vi "manage breakdown sub.vi"(8 "error in (no error)":errorcluster) -> (0 "error out":errorcluster)   [LabVIEW 2017]
uses:
  <vilib>/addons/database/Connection.llb/DB Tools Open Connec (Path).vi
  <vilib>/addons/database/NI_Database_API.lvlib
panel:
  in  "Action Related To":string(combo)
  in  "Expected Time To Close Action":string
  in  "Submit 2":bool
  in  "Get Reason  2":bool
  in  "CANCEL":bool
  in  "ID":string
  out "Table":string[][][](array[string])
  out "element":string
  out "index of element":i32
  out "data 2":string[][](array[string])
  in  "Select Reason":string(combo)
  in  "Add Action Taken":string
  in  "Shift":string(combo)
  in  "Select Station":string(combo)
  in  "Date":timestamp format="%<%Y-%m-%d>T"
  in  "Select Stakeholder":string(combo)
  # "Manage Breakdown"
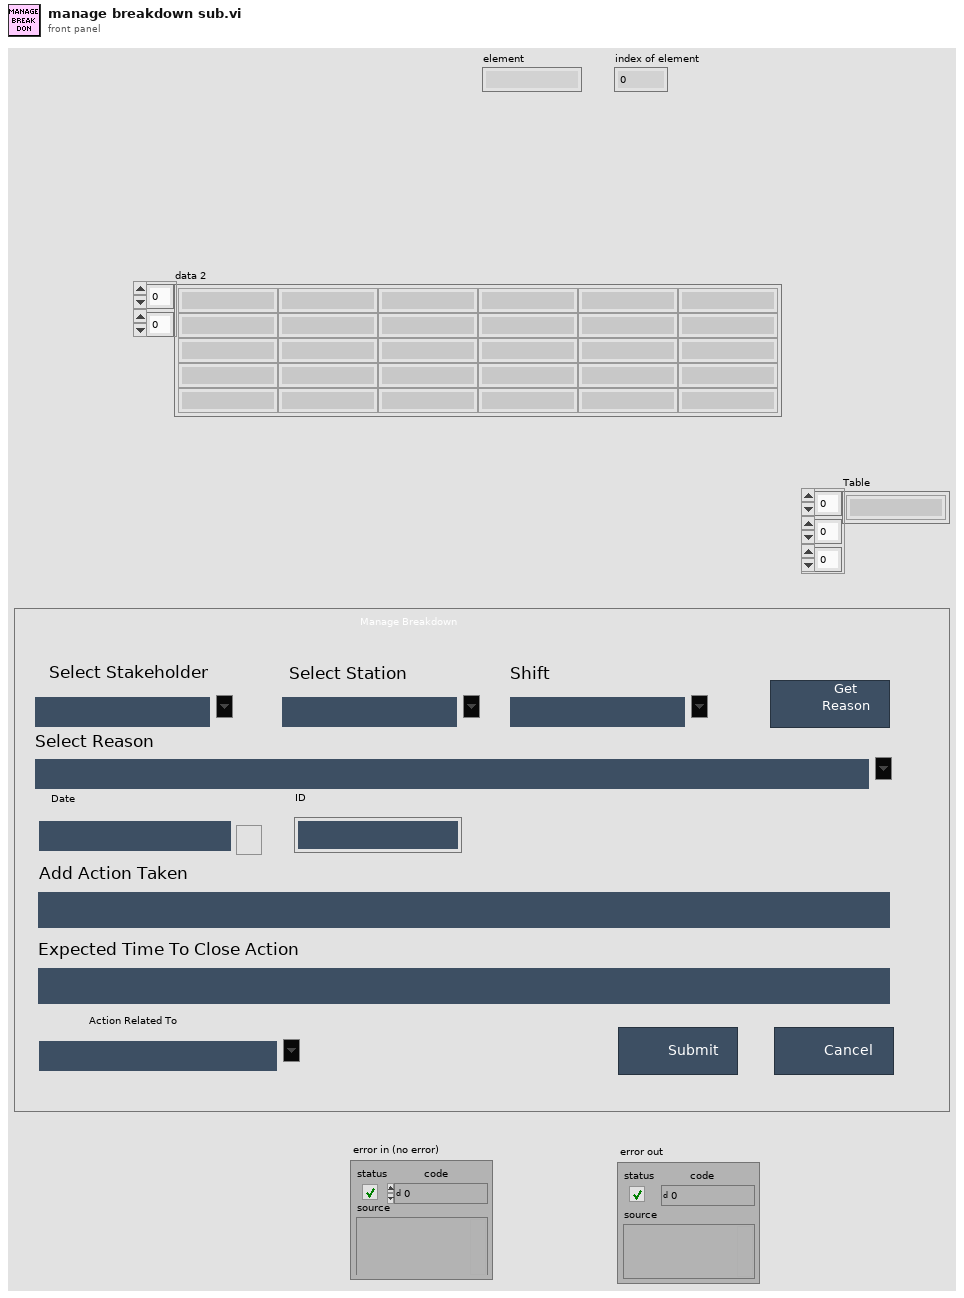
[diagram p1: front panel]
types:
  T1 = typedef "NI_Database_API.lvlib/Conn ObjectReference.ctl" = refnum<k1>
  T2 = enum32{"invalid app kind", "Development System", "Run Time System", "Student Edition", "Embedded LabVIEW", "Evaluation", "Custom"}
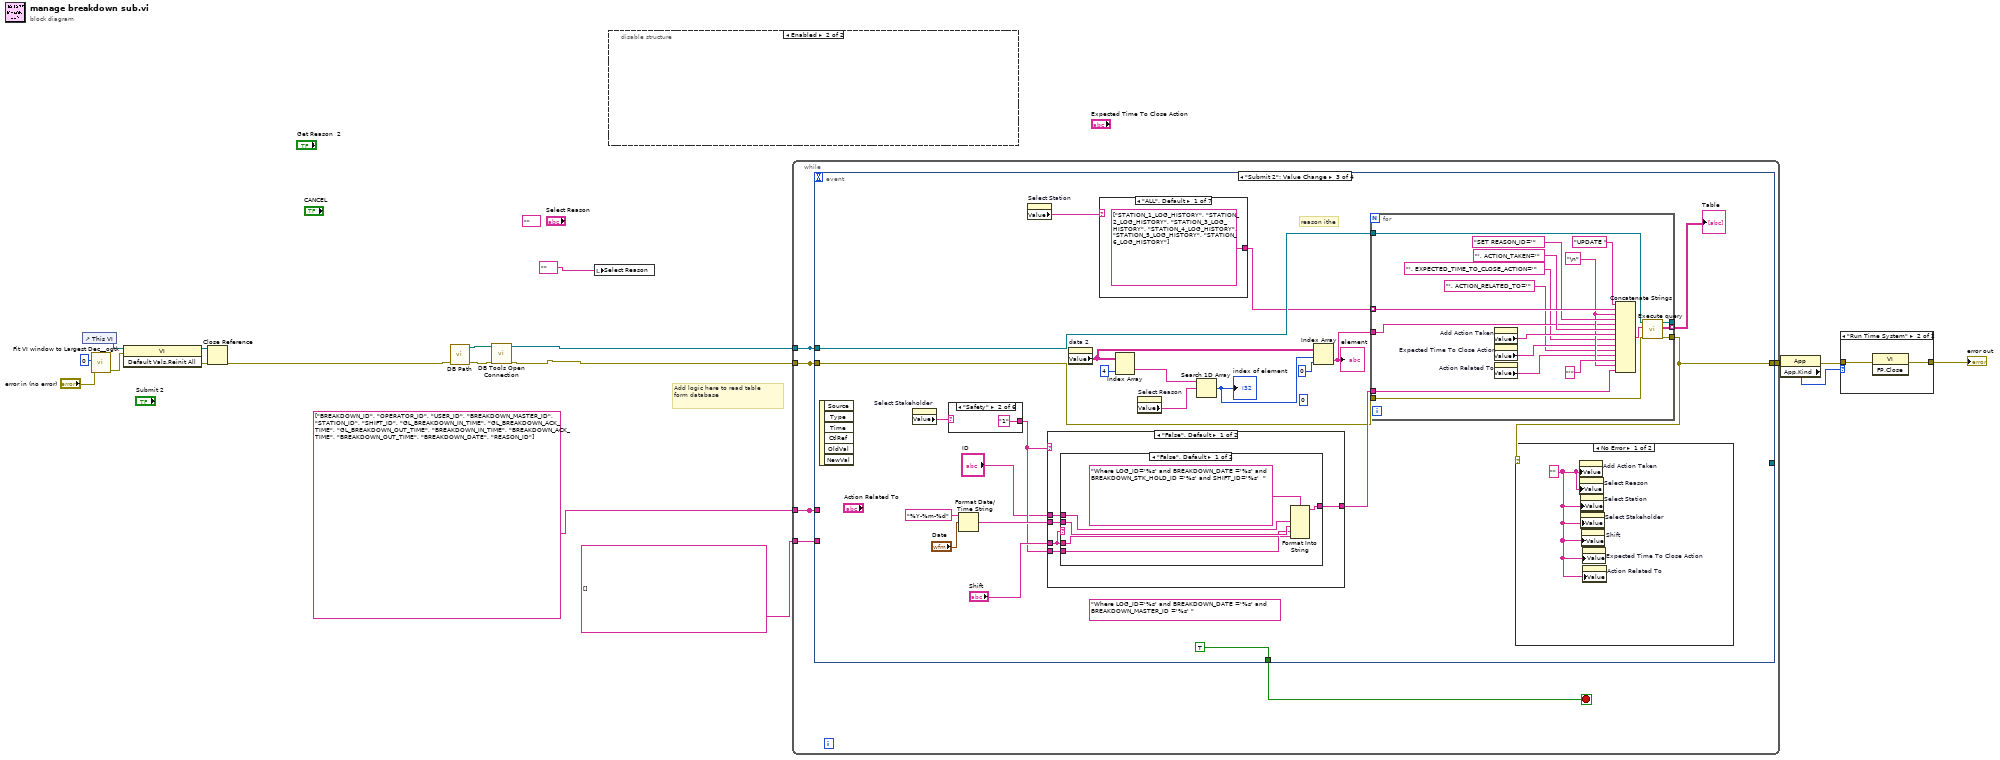
[diagram p0: block diagram]
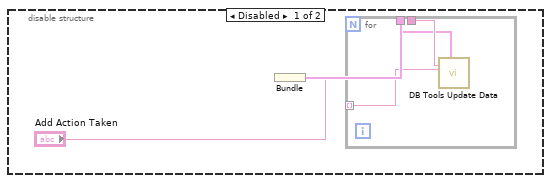
[diagram p2: hidden frame]
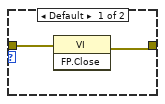
[diagram p3: hidden frame]
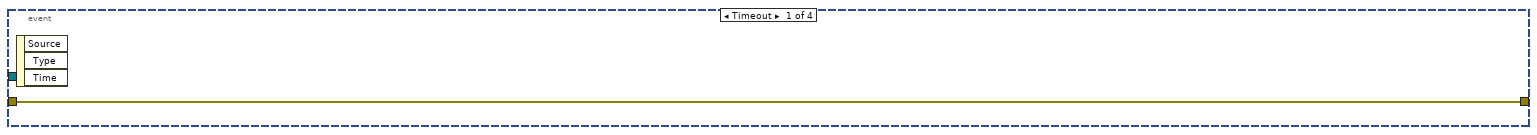
[diagram p4: hidden frame]
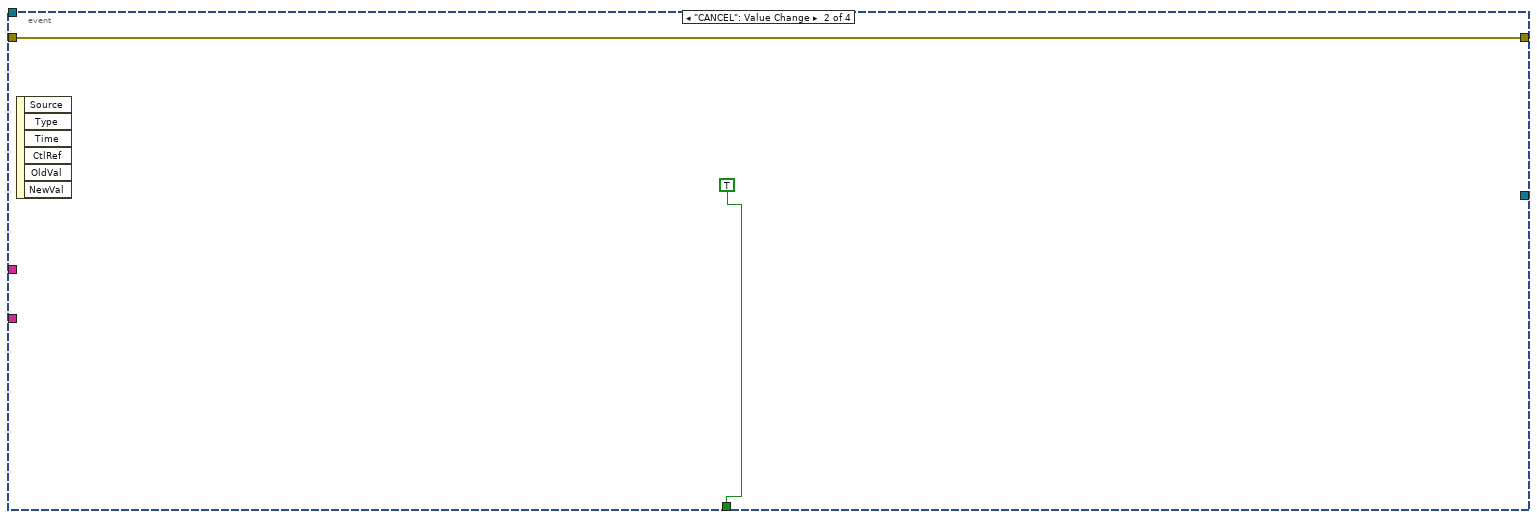
[diagram p5: hidden frame]
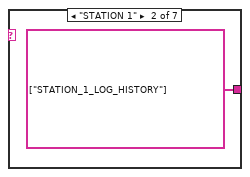
[diagram p6: hidden frame]
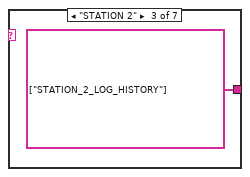
[diagram p7: hidden frame]
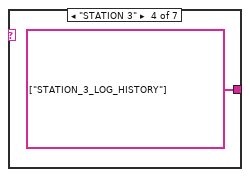
[diagram p8: hidden frame]
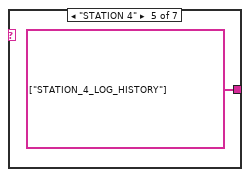
[diagram p9: hidden frame]
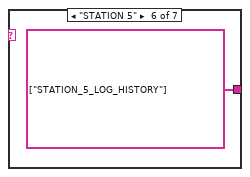
[diagram p10: hidden frame]
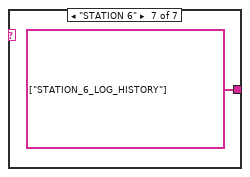
[diagram p11: hidden frame]
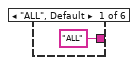
[diagram p13: hidden frame]
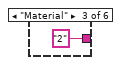
[diagram p14: hidden frame]
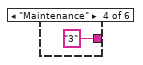
[diagram p15: hidden frame]
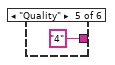
[diagram p16: hidden frame]
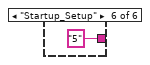
[diagram p17: hidden frame]
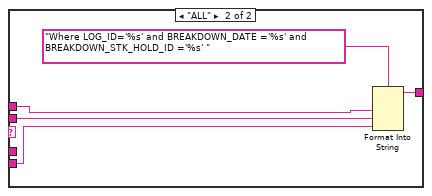
[diagram p18: hidden frame]
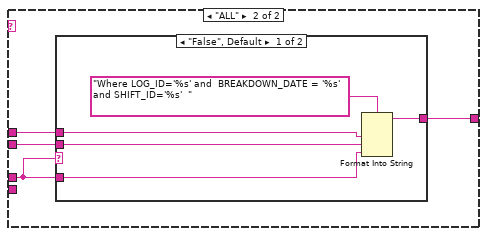
[diagram p19: hidden frame]
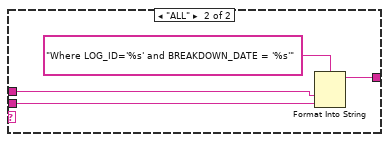
[diagram p20: hidden frame]
diagram:
  (unwired) "" ("Select Reason")
  # "Add logic here to read table\nform database"
  n1 = control-ref of="This VI"() -> (w18:refnum<vi>)
  n2 = call <userlib>:"Fit VI window to Largest Dec__ogtk.vi"("error in (no error)"="error in (no error)", "border spacing (2 px)"=0) -> ("error out"=w10:errorcluster)  [unwired: 4 in, 1 out]
  n3 = invoke class="VI" method="Default Vals.Reinit All"(reference=w18, error in=w10) -> (reference out=w16:refnum<vi>, error out=w17:errorcluster)  [unwired: 1 in, 1 out]
  n4 = Close Reference(reference=w16, error in (no error)=w17) -> (error out=w8:errorcluster)
  n5 = call "DB Path.vi"("error in"=w8) -> ("error out"=w6:errorcluster, "DB Path"=w7:path)  [unwired: 9 in]
  n6 = call-poly <vilib>:"DB Tools Open Connection.vi"("error in (no error)"=w6, "connection information"=w7) -> ("error out"=w5:errorcluster, "connection reference"=w4:T1)  [unwired: 6 in]
  n7 = local write "Select Reason"("" ("Combo Box")) -> ()
  n8 = disable-structure shown="Enabled" {
    frame Disabled {
      n9 = Bundle("Add Action Taken"="Add Action Taken") -> (w20:cluster{"Add Action Taken":string})  [unwired: 1 in]
      n10 = for {
        tunnel: _ -> [w23]
        tunnel: _ -> [w22] mode=indexing
        tunnel: w20 -> [w21]
        n11 = call <vilib>:"DB Tools Update Data.vi"("condition"=w23, "data"=w21, "table"=w22) -> ()  [unwired: 7 in, 2 out]
      }
    }
    frame Enabled {
    }
  }
  n12 = while {
    tunnel: w5 -> [w26]
    tunnel: [w24] -> w12
    tunnel: w4 -> [w27]
    tunnel: string[] ["BREAKDOWN_ID", "OPERATOR_ID", "USER_ID", "BREAKDOWN_MASTER_ID", "STATION_ID", "SHIFT_ID", "GL_BREAKDOWN_IN_TIME", "GL_BREAKDOWN_ACK_TIME", "GL_BREAKDOWN_OUT_TIME", "BREAKDOWN_IN_TIME", "BREAKDOWN_ACK_TIME", "BREAKDOWN_OUT_TIME", "BREAKDOWN_DATE", "REASON_ID"] ("columns") -> [w28]
    tunnel: [w28] -> _
    tunnel: [w26] -> _
    tunnel: [w27] -> _
    tunnel: string[] [] -> [w25]
    stop <- w29 stop-if-true
    n13 = event shown="[2] \"Submit 2\": Value Change" {
      selector: _ -> [_ _ _ _]
      dyn-events: _ -> [_ _ _ _]
      timeout: _ -> [_ _ _ _]
      tunnel: [_ TRUE TRUE _] -> w29
      tunnel: w27 -> [_ _ w40 w131]
      tunnel: w28 -> [_ _ _ _]
      tunnel: w26 -> [w30 w32 w41 w130]
      tunnel: [_ _ _ w129] -> _
      tunnel: w25 -> [_ _ _ _]
      tunnel: [w30 w32 w36 w122] -> w24
      event Timeout {
        n14 = event-data() -> ()  [unwired: 1 in, 3 out]
      }
      event "CANCEL": Value Change {
        n15 = event-data() -> ()  [unwired: 1 in, 6 out]
      }
      event "Submit 2": Value Change {
        (unwired) "Where LOG_ID='%s' and BREAKDOWN_DATE ='%s' and BREAKDOWN_MASTER_ID ='%s' " ("condition")
        (unwired) 0 ("disabled index (col)")
        # "reason ithe"
        n16 = event-data() -> ()  [unwired: 1 in, 6 out]
        n17 = property on="Select Stakeholder" class="CmbBox"() -> ("Value"=w39:string)  [unwired: 2 in, 2 out]
        n18 = case shown="\"Safety\"" w39 {
          tunnel: ["ALL" "1" "2" "3" "4" "5"] -> w38
          frame "ALL", Default {
          }
          frame "Safety" {
          }
          frame "Material" {
          }
          frame "Maintenance" {
          }
          frame "Quality" {
          }
          frame "Startup_Setup" {
          }
        }
        n19 = Format Date/Time String(time format string (%c)="%Y-%m-%d", seconds (now)="Date") -> (date/time string=w47:string)  [unwired: 1 in]
        n20 = property on="Select Station" class="CmbBox"() -> ("Value"=w34:string)  [unwired: 2 in, 2 out]
        n21 = case shown="\"False\", Default" w38 {
          tunnel: [w92 w107] -> w48
          tunnel: w47 -> [w91 w106]
          tunnel: w38 -> [w90 _]
          tunnel: "Shift" -> [w89 w105]
          tunnel: "ID" -> [w88 w104]
          frame "False", Default {
            n22 = case shown="\"False\", Default" w89 {
              tunnel: [w97 w102] -> w92
              tunnel: w91 -> [w96 w101]
              tunnel: w90 -> [w95 w100]
              tunnel: w89 -> [w94 _]
              tunnel: w88 -> [w93 w99]
              frame "False", Default {
                n23 = Format Into String(format string="Where LOG_ID='%s' and BREAKDOWN_DATE ='%s' and BREAKDOWN_STK_HOLD_ID ='%s' and SHIFT_ID='%s'  " ("condition"), w93, w96, w95, w94) -> (resulting string=w97:string)  [unwired: 2 in, 1 out]
              }
              frame "ALL" {
                n24 = Format Into String(format string="Where LOG_ID='%s' and BREAKDOWN_DATE ='%s' and BREAKDOWN_STK_HOLD_ID ='%s' " ("condition"), w99, w101, w100) -> (resulting string=w102:string)  [unwired: 2 in, 1 out]
              }
            }
          }
          frame "ALL" {
            n25 = case shown="\"False\", Default" w105 {
              tunnel: [w111 w115] -> w107
              tunnel: w106 -> [w110 w114]
              tunnel: w105 -> [w109 _]
              tunnel: w104 -> [w108 w113]
              frame "False", Default {
                n26 = Format Into String(format string="Where LOG_ID='%s' and  BREAKDOWN_DATE = '%s' and SHIFT_ID='%s'  " ("condition"), w108, w110, w109) -> (resulting string=w111:string)  [unwired: 2 in, 1 out]
              }
              frame "ALL" {
                n27 = Format Into String(format string="Where LOG_ID='%s' and BREAKDOWN_DATE = '%s'" ("condition"), w113, w114) -> (resulting string=w115:string)  [unwired: 2 in, 1 out]
              }
            }
          }
        }
        n28 = property on="data 2" class="Arr (strict)"() -> ("Value"=w51:string[][])  [unwired: 2 in, 2 out]
        n29 = case shown="\"ALL\", Default" w34 {
          tunnel: [string[] ["STATION_1_LOG_HISTORY", "STATION_2_LOG_HISTORY", "STATION_3_LOG_HISTORY", "STATION_4_LOG_HISTORY", "STATION_5_LOG_HISTORY", "STATION_6_LOG_HISTORY"] string[] ["STATION_1_LOG_HISTORY"] string[] ["STATION_2_LOG_HISTORY"] string[] ["STATION_3_LOG_HISTORY"] string[] ["STATION_4_LOG_HISTORY"] string[] ["STATION_5_LOG_HISTORY"] string[] ["STATION_6_LOG_HISTORY"]] -> w33
          frame "ALL", Default {
          }
          frame "STATION 1" {
          }
          frame "STATION 2" {
          }
          frame "STATION 3" {
          }
          frame "STATION 4" {
          }
          frame "STATION 5" {
          }
          frame "STATION 6" {
          }
        }
        n30 = Index Array(array=w51, index (col)=4 ("disabled index (col)")) -> (element=w49:string[])  [unwired: 1 in]
        n31 = property on="Select Reason" class="CmbBox"() -> ("Value"=w52:string)  [unwired: 2 in, 2 out]
        n32 = Search 1D Array(1D array=w49, element=w52) -> (index of element=w50:i32)  [unwired: 1 in]
        "index of element" <- w50
        n33 = Index Array(array=w51, index (row)=w50, index (col)=0 ("disabled index (col)")) -> (element=w53:string)
        "element" <- w53
        n34 = for {
          tunnel: w33 -> [w85] mode=indexing
          tunnel: w48 -> [w79]
          tunnel: w53 -> [w78]
          tunnel: [w77] -> _
          tunnel: w40 -> [w76]
          tunnel: [w75] -> w36
          tunnel: w41 -> [w74]
          tunnel: [w73] -> w37 mode=indexing
          w80 = "\n" ("string")
          n35 = property on="Add Action Taken" class="Str"() -> ("Value"=w82:string)  [unwired: 2 in, 2 out]
          n36 = property on="Expected Time To Close Action" class="Str"() -> ("Value"=w71:string)  [unwired: 2 in, 2 out]
          n37 = property on="Action Related To" class="CmbBox"() -> ("Value"=w69:string)  [unwired: 2 in, 2 out]
          n38 = Concatenate Strings("UPDATE " ("String"), w85, w80, "SET REASON_ID='" ("string"), w78, "', ACTION_TAKEN='" ("string"), w82, "', EXPECTED_TIME_TO_CLOSE_ACTION='" ("string"), w71, "', ACTION_RELATED_TO='" ("string"), w69, "'" ("string"), w80, w79) -> (w86:string)
          n39 = call "Execute query.vi"("error in (no error)"=w74, "String"=w86, "connection reference"=w76) -> ("error out"=w75:errorcluster, "Table"=w73:string[][], "connection reference 2"=w77:T1)  [unwired: 3 in, 3 out]
        }
        "Table" <- w37
        n40 = case shown="No Error" w36 {
          frame No Error {
            w62 = ""
            n41 = property on="Add Action Taken" class="Str"("Value"=w62) -> ()  [unwired: 2 in, 2 out]
            n42 = property on="Select Reason" class="CmbBox"("Value"=w62) -> ()  [unwired: 2 in, 2 out]
            n43 = property on="Select Station" class="CmbBox"("Value"=w62) -> ()  [unwired: 2 in, 2 out]
            n44 = property on="Select Stakeholder" class="CmbBox"("Value"=w62) -> ()  [unwired: 2 in, 2 out]
            n45 = property on="Shift" class="CmbBox"("Value"=w62) -> ()  [unwired: 2 in, 2 out]
            n46 = property on="Expected Time To Close Action" class="Str"("Value"=w62) -> ()  [unwired: 2 in, 2 out]
            n47 = property on="Action Related To" class="CmbBox"("Value"=w62) -> ()  [unwired: 2 in, 2 out]
          }
          frame Error {
          }
        }
      }
      event "Get Reason  2": Value Change {
        (unwired) string[] ["1", "2", "3", "4", "5", "6", "7", "8", "9", "10", "11", "12", "13", "14", "15", "16", "17", "18", "19", "20", "21", "22", "23"]
        n48 = event-data() -> ()  [unwired: 1 in, 6 out]
        n49 = case shown="\"STATION 1\"" "Select Station" {
          tunnel: [string[] ["1", "2", "3", "4", "5", "6"] string[] ["1"] string[] ["2"] string[] ["3"] string[] ["4"] string[] ["5"] string[] ["6"] string[] ["7"] string[] ["8"] string[] ["9"] string[] ["10"] string[] ["11"] string[] ["12"] string[] ["13"] string[] ["14"] string[] ["15"] string[] ["16"] string[] ["17"] string[] ["18"] string[] ["19"] string[] ["20"] string[] ["21"] string[] ["22"] string[] ["23 "]] -> w127
          frame "ALL", Default {
          }
          frame "STATION 1" {
          }
          frame "STATION 2" {
          }
          frame "STATION 3" {
          }
          frame "STATION 4" {
          }
          frame "STATION 5" {
          }
          frame "STATION 6" {
          }
          frame "HVI" {
          }
          frame "7009" {
          }
          frame "SA" {
          }
          frame "M&M" {
          }
          frame "TML" {
          }
          frame "5001" {
          }
          frame "1001" {
          }
          frame "4003" {
          }
          frame "1002" {
          }
          frame "4004" {
          }
          frame "1004" {
          }
          frame "2001" {
          }
          frame "3001" {
          }
          frame "2004" {
          }
          frame "3002" {
          }
          frame "3003" {
          }
          frame "4001" {
          }
        }
        n50 = case shown="\"Material\"" "Select Stakeholder" {
          tunnel: ["ALL" "1" "2" "3" "4" "5"] -> w117
          frame "ALL", Default {
          }
          frame "Safety" {
          }
          frame "Material" {
          }
          frame "Maintenance" {
          }
          frame "Quality" {
          }
          frame "Startup_Setup" {
          }
        }
        n51 = for {
          tunnel: w127 -> [w143] mode=indexing
          tunnel: w130 -> [w147]
          tunnel: [w144] -> w123
          tunnel: w131 -> [w148]
          tunnel: [w145] -> w129
          tunnel: w117 -> [w142]
          shift-right: [w138] -> w125
          shift-left: variant[][] [] -> [w139]
          n52 = case shown="\"ALL\"" w142 {
            tunnel: [w152 w154] -> w146
            tunnel: w143 -> [w150 w153]
            tunnel: w142 -> [w149 _]
            frame "False", Default {
              n53 = Format Into String(format string="Where STATION_ID ='%s' and BREAKDOWN_MASTER_ID ='%s' " ("condition"), w150, w149) -> (resulting string=w152:string)  [unwired: 2 in, 1 out]
            }
            frame "ALL" {
              n54 = Format Into String(format string="Where STATION_ID = '%s'" ("condition"), w153) -> (resulting string=w154:string)  [unwired: 2 in, 1 out]
            }
          }
          n55 = call <vilib>:"DB Tools Select Data.vi"("condition"=w146, "error in (no error)"=w147, "table"="master_reason", "connection reference"=w148) -> ("error out"=w144:errorcluster, "data"=w140:variant[][], "connection reference out"=w145:T1)  [unwired: 2 in]
          n56 = Build Array (concatenate)(w139, w140) -> (w138:variant[][])
        }
        n57 = Variant To Data(error in=w123, type=string[][] [], Variant=w125) -> (data=w121:string[][], error out=w122:errorcluster)
        "data 2" <- w121
        n58 = Index Array(array=w121, index (col)=4 ("disabled index (col)")) -> (element=w119:string[])  [unwired: 1 in]
        n59 = property on="Select Reason" class="CmbBox"("Strings[]"=w119) -> ()  [unwired: 2 in, 2 out]
      }
    }
  }
  n60 = property class="App"(error in=w12) -> (error out=w14:errorcluster, "App.Kind"=w15:T2)  [unwired: 1 in, 1 out]
  n61 = case shown="\"Run Time System\"" w15 {
    tunnel: w14 -> [w181 w183]
    tunnel: [w180 w182] -> w13
    frame Default {
      n62 = invoke class="VI" method="FP.Close"(error in=w181) -> (error out=w180:errorcluster)  [unwired: 2 in, 2 out]
    }
    frame "Run Time System" {
      n63 = invoke class="VI" method="FP.Close"(error in=w183) -> (error out=w182:errorcluster)  [unwired: 2 in, 2 out]
    }
  }
  "error out" <- w13
